vi "Transmitter_TDMA - With Timer.vi"() -> ()   [LabVIEW 2022 SP3]
uses:
  <instrlib>/niUSRP/niUSRP Write Tx Data (CDB).vi
panel:
  in  "Data bit length":i32
  in  "Iterations":i32=10000
  out "Time(s)":sgl format="%#_4g"
  in  "Alpha":dbl(slide)=0.17500000000000002 step=0.005 scale=0.0..1.0
  in  "Tab Control":enum32{"USRP Parameters", "Transmission"}(tab)
  in  "USRP ControledParameters 2":T1={"Active Antenna"="TX1", "Gain (dB)"=0.0, "Carrier Frequency"=2400000000.0, "IQ Rate"=2000000.0, "Active Channel"="0"} {"IQ Rate" format="%#_6p"; "Carrier Frequency" format="%#_6p"; "Gain (dB)" format="%#_6f"}
  in  "Device selection":refnum<k15>="RIO0"
  in  "stop":bool
  out "Error out":errorcluster
  in  "Modulation parameter":T2
  out "Bits length":i32
  out "Bits length 2":i32
  out "Frame Duration":dbl format="%#_6p"
  out "Coerced Parameters":T3={"IQ Rate"=100000.0, "Carrier  Freq."=100000.0, "Gain"=0.0} {"Gain" format="%#_6f"; "Carrier  Freq." format="%#_6p"; "IQ Rate" format="%#_6p"}
  out "Transmitted Waveform":dbl[](graph)
  in  "Message 2":string="ptua. At vero eos et accusam et justo duo dolores et ea rebum. Stet clita kasd gubergren, no sea takimata sanctus est Lorem ipsum dolor sit amet. Lore"
  in  "Message 1":string="Lorem ipsum dolor sit amet, consetetur sadipscing elitr, sed diam nonumy eirmod tempor invidunt ut labore et dolore magna aliquyam erat, sed diam volu"
  in  "error in (no error)":errorcluster
  # "RSMA Transmitter"
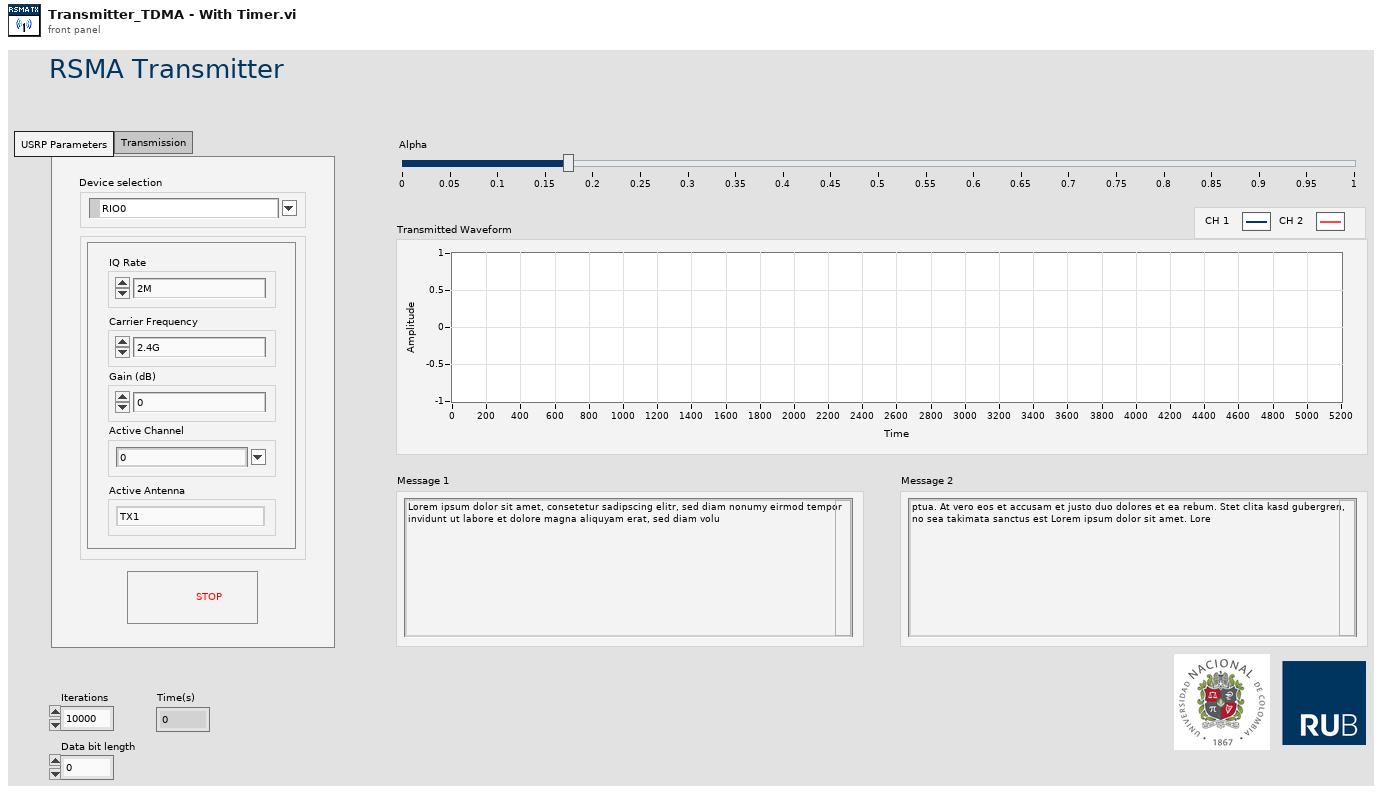
[diagram p1: front panel]
types:
  T1 = cluster{"Active Antenna":string, "Gain (dB)":dbl, "Carrier Frequency":dbl, "IQ Rate":dbl, "Active Channel":string}
  T2 = cluster{"Modulation type":enum16{"QPSK(4QAM)", "64QAM", "16QAM", "BPSK"}, "BCC rate (k/n)":enum16{"1/2", "2/3", "3/4"}}
  T3 = cluster{"IQ Rate":dbl, "Carrier  Freq.":dbl, "Gain":dbl}
  T4 = cluster{"coerced IQ rate":dbl, "coerced carrier frequency":dbl, "coerced gain":dbl}
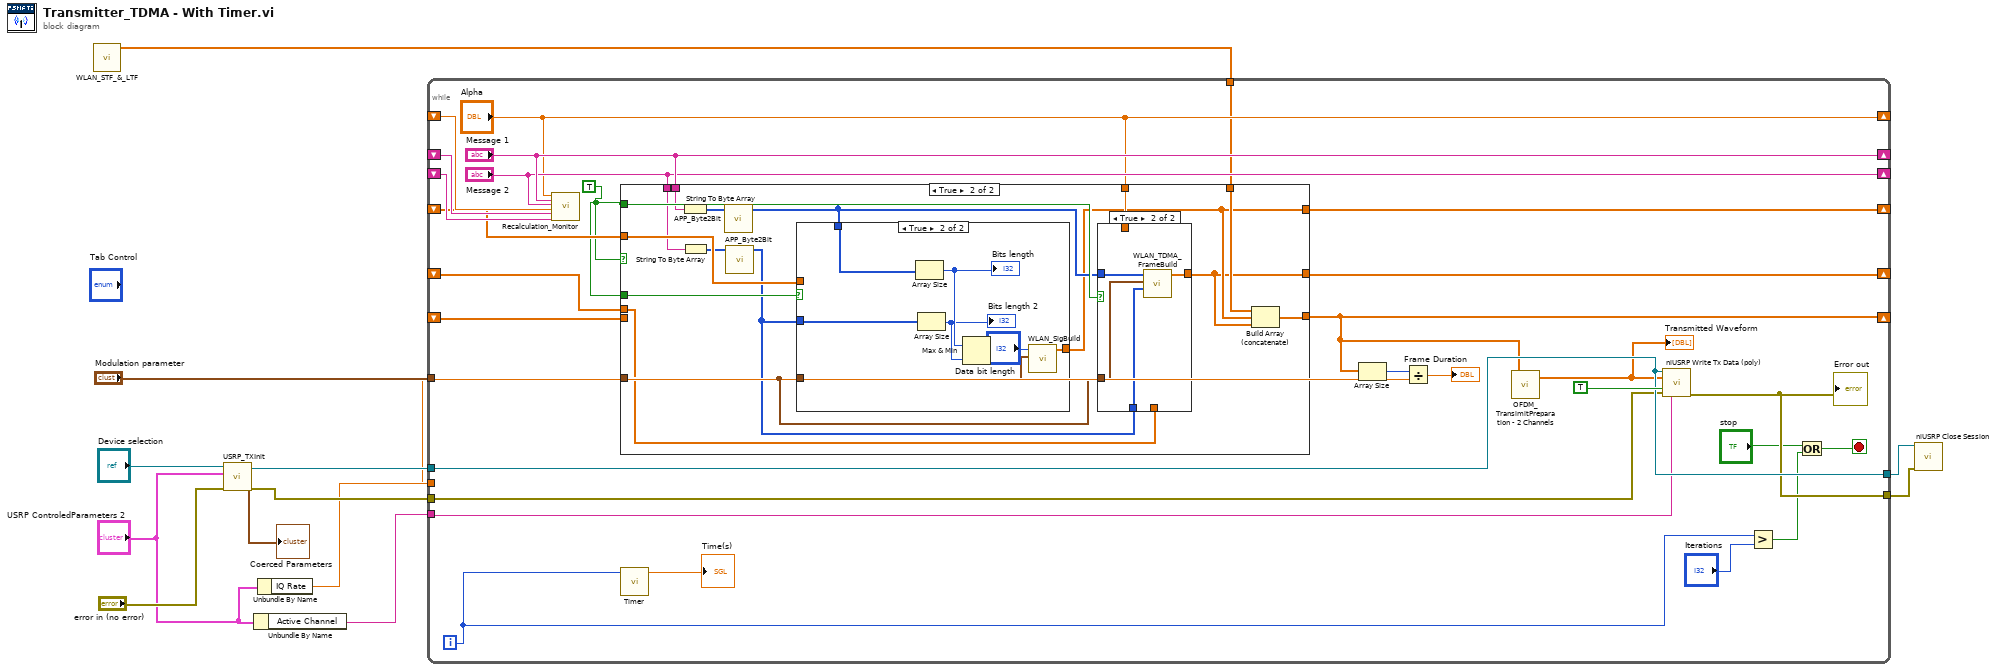
[diagram p0: block diagram]
diagram:
  n1 = call "WLAN_STF_&_LTF.vi"() -> ("STF & LTF"=w1:cdb[])  [unwired: 11 in]
  n2 = call "USRP_TXInit.vi"("device names"="Device selection", "USRP ControledParameters"="USRP ControledParameters 2", "error in (no error)"="error in (no error)") -> ("session handle out"=w11:refnum<k15>, "USRP CoercedParamters"=→"Coerced Parameters":T4, "error out"=w10:errorcluster)  [unwired: 5 in]
  n3 = Unbundle By Name("USRP ControledParameters 2") -> ("Active Channel"=w3:string)
  n4 = Unbundle By Name("USRP ControledParameters 2") -> ("IQ Rate"=w9:dbl)
  n5 = while {
    tunnel: w11 -> [w39]
    tunnel: w10 -> [w22]
    tunnel: w9 -> [w38]
    tunnel: [w39] -> w8
    tunnel: [w37] -> w7
    tunnel: w3 -> [w36]
    shift-right: ["Alpha"] -> _
    shift-left: _ -> [w35]
    shift-right: ["Message 1"] -> _
    shift-left: _ -> [w34]
    shift-right: ["Message 2"] -> _
    shift-left: _ -> [w33]
    tunnel: "Modulation parameter" -> [w30]
    shift-right: [w29] -> _
    shift-left: _ -> [w28]
    shift-right: [w26] -> _
    shift-left: _ -> [w25]
    tunnel: w1 -> [w24]
    shift-right: [w21] -> _
    shift-left: _ -> [w23]
    i -> [w17]
    stop <- w14 stop-if-true
    w13 = TRUE
    n6 = call "Recalculation_Monitor.vi"("Alpha"="Alpha", "Message 1"="Message 1", "Message 2"="Message 2", "Alpha old"=w35, "Message 1 old"=w34, "Message 2 old"=w33) -> ()  [unwired: 11 in, 3 out]
    n7 = case shown="True" w13 {
      tunnel: w13 -> [_ w61]
      tunnel: w13 -> [_ w60]
      tunnel: "Message 1" -> [_ w55]
      tunnel: "Message 2" -> [_ w56]
      tunnel: w30 -> [_ w52]
      tunnel: [w45 w48] -> w29
      tunnel: w28 -> [w45 w59]
      tunnel: "Alpha" -> [_ w51]
      tunnel: [w44 w47] -> w26
      tunnel: w25 -> [w44 w50]
      tunnel: w24 -> [_ w49]
      tunnel: [w43 w46] -> w21
      tunnel: w23 -> [w43 _]
      frame False {
      }
      frame True {
        n8 = String To Byte Array(string=w55) -> (unsigned byte array=w57:u8[])
        n9 = String To Byte Array(string=w56) -> (unsigned byte array=w58:u8[])
        n10 = call "APP_Byte2Bit.vi"("input byte stream"=w57) -> ("output bit stream"=w53:i8[])  [unwired: 10 in]
        n11 = call "APP_Byte2Bit.vi"("input byte stream"=w58) -> ("output bit stream"=w54:i8[])  [unwired: 10 in]
        n12 = case shown="True" w61 {
          tunnel: w52 -> [_ w69]
          tunnel: [w67 w72] -> w48
          tunnel: w59 -> [w67 _]
          tunnel: w54 -> [_ w71]
          tunnel: w53 -> [_ w70]
          frame False {
          }
          frame True {
            n13 = Array Size(array=w70) -> (size(s)=w74:i32)
            "Bits length" <- w74
            n14 = Array Size(array=w71) -> (size(s)=w73:i32)
            "Bits length 2" <- w73
            n15 = Max & Min(x=w74, y=w73) -> ()  [unwired: 2 out]
            n16 = call "WLAN_SigBuild.vi"("Data bit length"="Data bit length", "Modulation parameter"=w69) -> ("symbols"=w72:cdb[])  [unwired: 7 in, 1 out]
          }
        }
        n17 = case shown="True" w60 {
          tunnel: w54 -> [_ w66]
          tunnel: w53 -> [_ w65]
          tunnel: w52 -> [_ w64]
          tunnel: w51 -> [_ _]
          tunnel: [w62 w63] -> w47
          tunnel: w50 -> [w62 _]
          frame False {
          }
          frame True {
            n18 = call "WLAN_TDMA_FrameBuild.vi"("data in 2"=w66, "Modulation parameter"=w64, "data in"=w65) -> ("output array"=w63:cdb[])  [unwired: 7 in, 1 out]
          }
        }
        n19 = Build Array (concatenate)(w49, w48, w47) -> (w46:cdb[])
      }
    }
    n20 = call "Timer.vi"("index"=w17) -> ("Time(s)"=→"Time(s)":sgl)  [unwired: 10 in]
    n21 = Array Size(array=w21) -> (size(s)=w41:i32)
    n22 = Divide(x=w41, y=w38) -> (x/y=→"Frame Duration":dbl)
    n23 = call "OFDM_TransimitPreparation - 2 Channels.vi"("array"=w21) -> ("output array"=w20:cdb[])  [unwired: 8 in, 2 out]
    "Transmitted Waveform" <- w20
    n24 = call-poly <instrlib>:"niUSRP Write Tx Data (poly).vi"("session handle"=w39, "channel list"=w36, "data"=w20, "end of data?"=TRUE, "error in (no error)"=w22) -> ("error out"=w37:errorcluster)  [unwired: 9 in, 1 out]
    "Error out" <- w37
    n25 = Greater?(x=w17, y="Iterations") -> (0:w15:bool)
    n26 = Or(x="stop", y=w15) -> (x .or. y?=w14:bool)
  }
  n27 = call <instrlib>:"niUSRP Close Session.vi"("session handle"=w8, "error in (no error)"=w7) -> ()  [unwired: 13 in, 1 out]
